vi "patientCreateView.vi"() -> ()   [LabVIEW 2019]
doc: "40"
uses:
  03_Home/controller/logoutBtn.ctl
  03_Home/controller/exitBtn.ctl
  <vilib>/Utility/miscctls.llb/LVPointTypeDef.ctl
  03_Home/controller/pannelState.ctl
  subVI/patients_state.ctl
  globalValue.vi
panel:
  in  "patients_weight":dbl format="%.1f"
  in  "patients_age":dbl
  in  "patients_height":dbl format="%.1f"
  in  "patients_birthdate":dbl format="%<%Y-%m-%d>T"
  in  "patients_gender":string(combo)
  in  "backPage":bool
  in  "patients_info":string
  in  "patients_address":string
  in  "patients_phone":string
  in  "patients_email":string
  in  "patients_nm":string
  in  "cancelBtn":bool
  in  "createBtn":bool
  out "patients_id":string
  in  "Help Button":bool
  in  "LogOut Button":T1
  in  "Exit Button":T2
  out "userNm":string
  # "|"
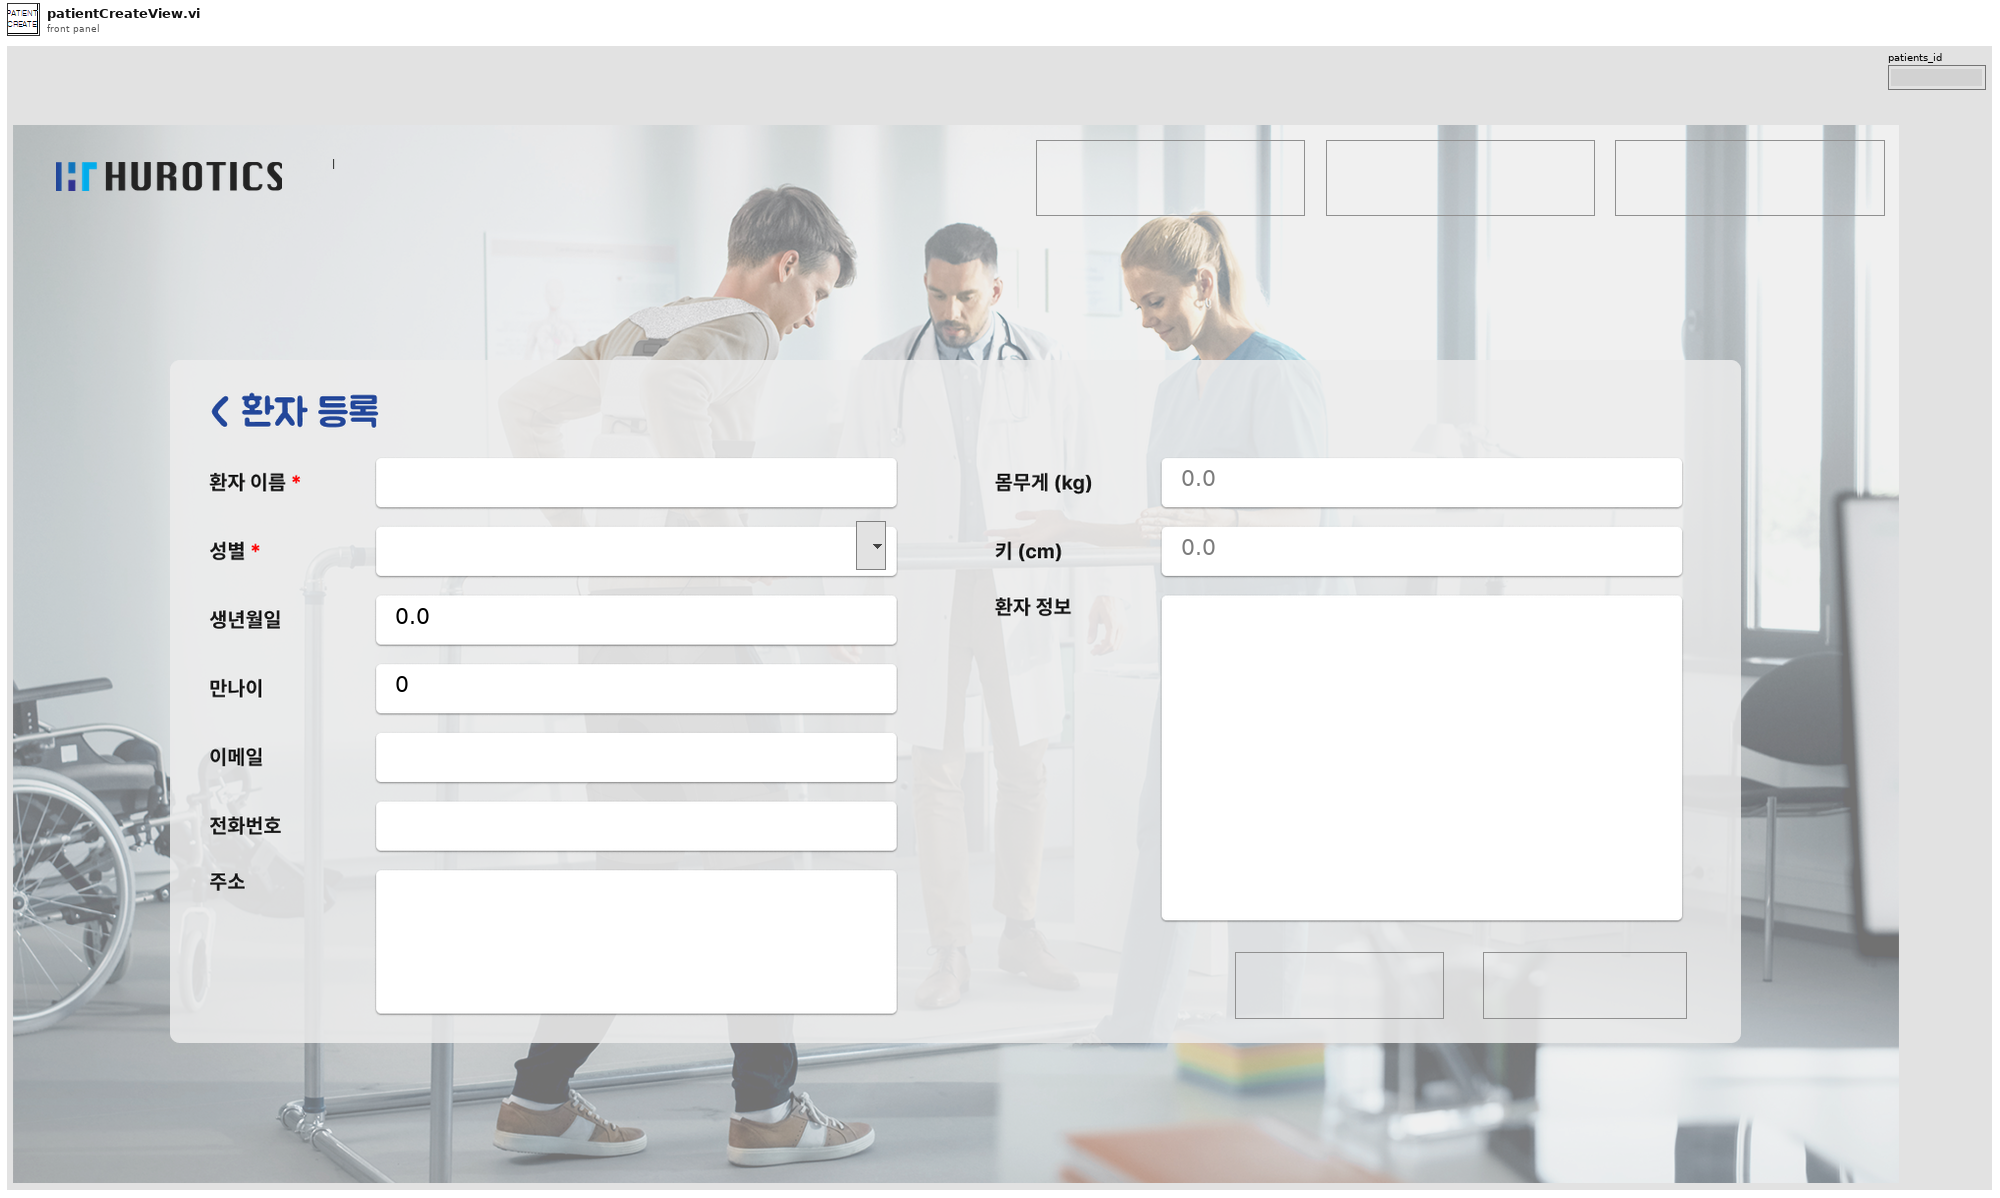
[diagram p1: front panel]
types:
  T1 = typedef "logoutBtn.ctl" = bool
  T2 = typedef "exitBtn.ctl" = bool
  T3 = typedef "LVPointTypeDef.ctl" = cluster{"Horizontal":i16, "Vertical":i16}
  T4 = enum16{"connection", "create", "getReadList", "getRead", "getCount", "update", "delete", "close"}
  T5 = typedef "pannelState.ctl" = enum16{"Init", "LogIn", "SignUpView", "Home", "Management_patientList", "Management_patientTrashtList", "Management_patientCreate", "Management_patientUpdate", "Management_patientTraining", "Management_patientTrainingDetail", "H-MEDI PatientList", "H-MEDI HardwareCtl", "Adjust", "FineTuning", "UserList", "UserDetail", "Exit"}
  T6 = typedef "patients_state.ctl" = enum16{"connection", "create", "getReadList", "getRead", "getCount", "update", "delete", "trash", "restore", "close"}
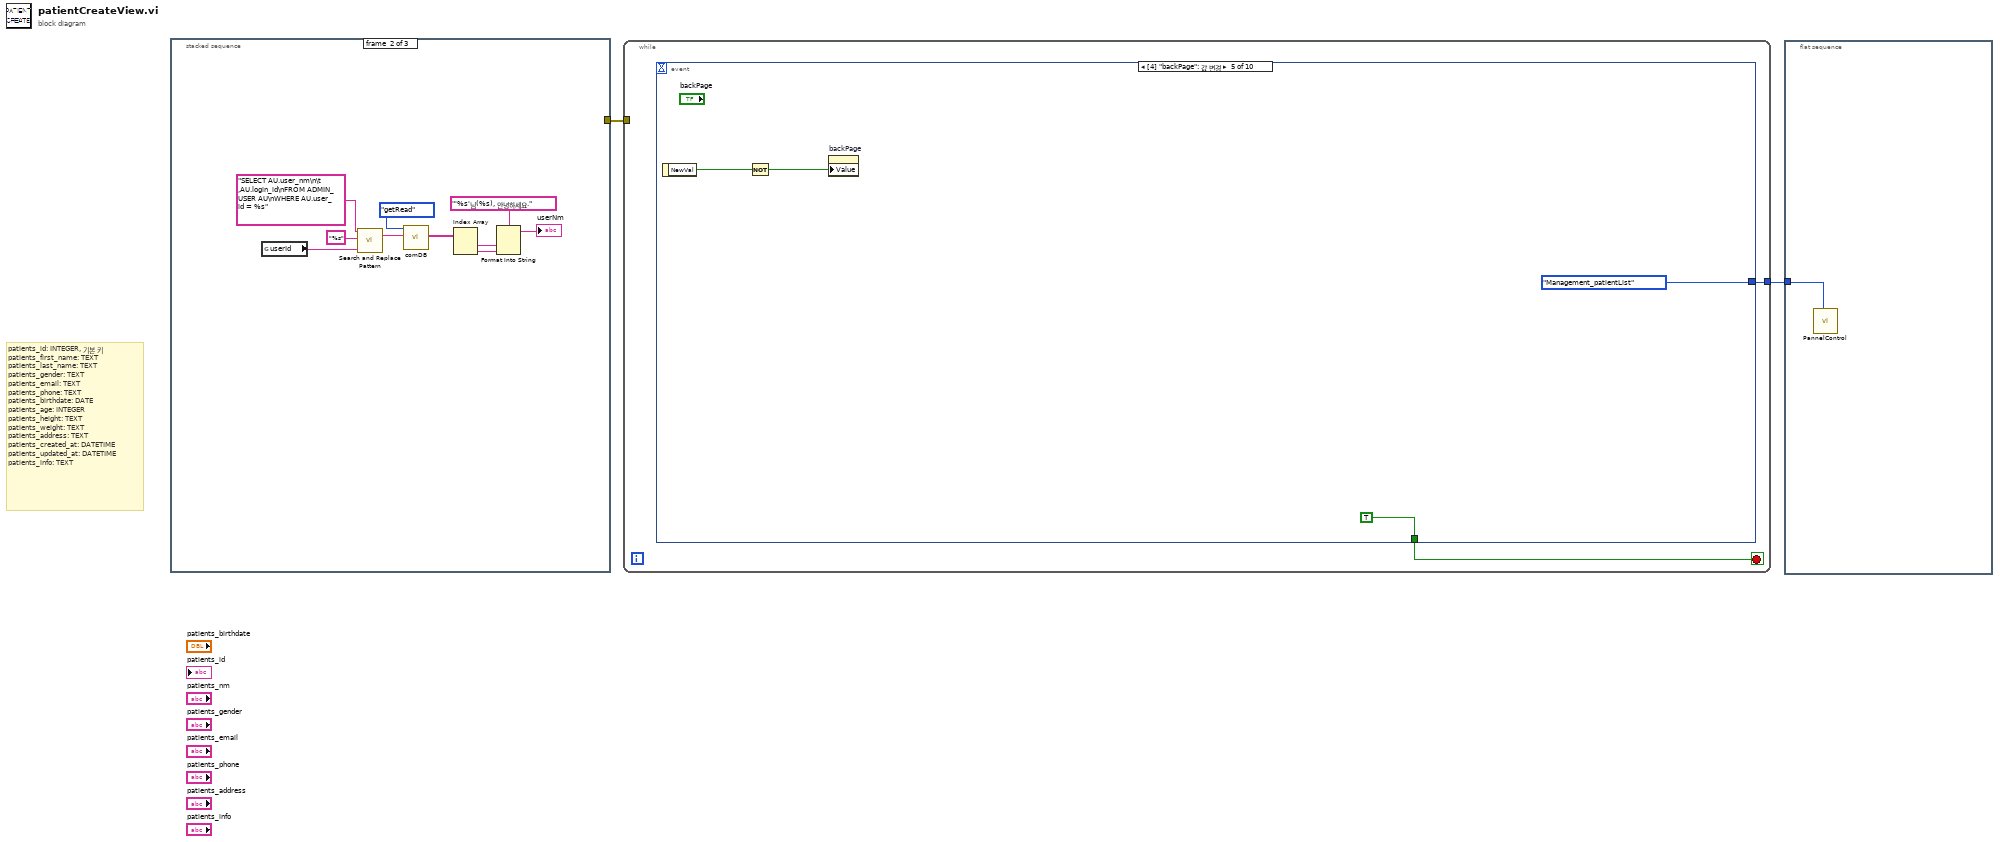
[diagram p0: block diagram]
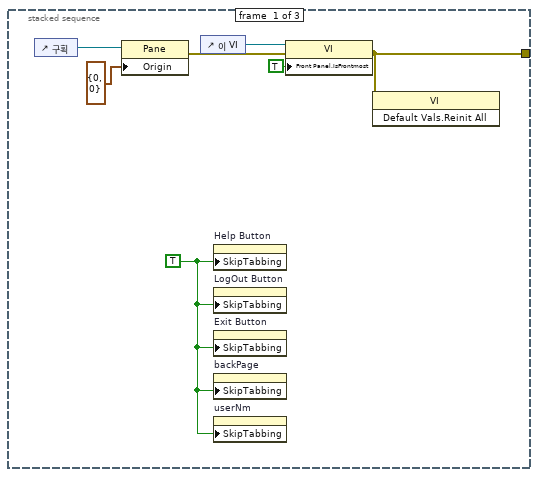
[diagram p2: hidden frame]
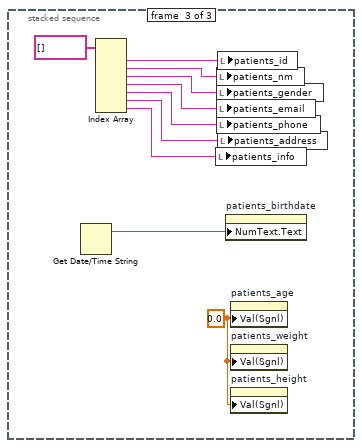
[diagram p3: hidden frame]
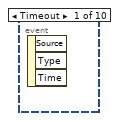
[diagram p4: hidden frame]
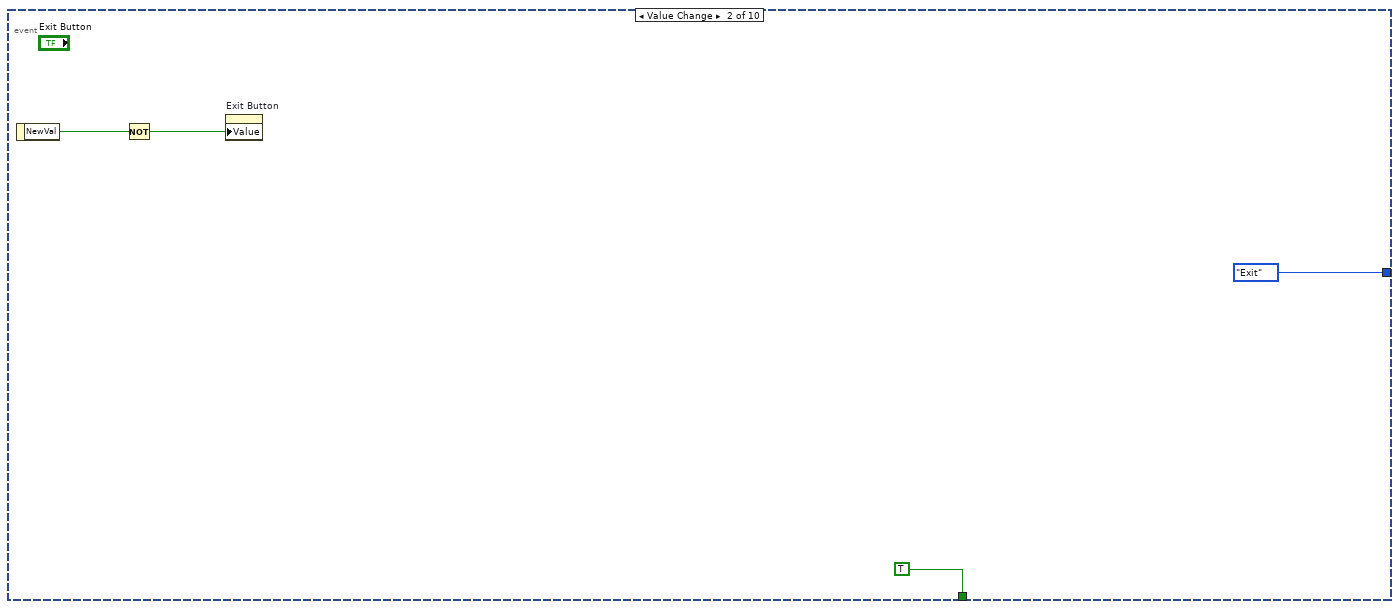
[diagram p5: hidden frame]
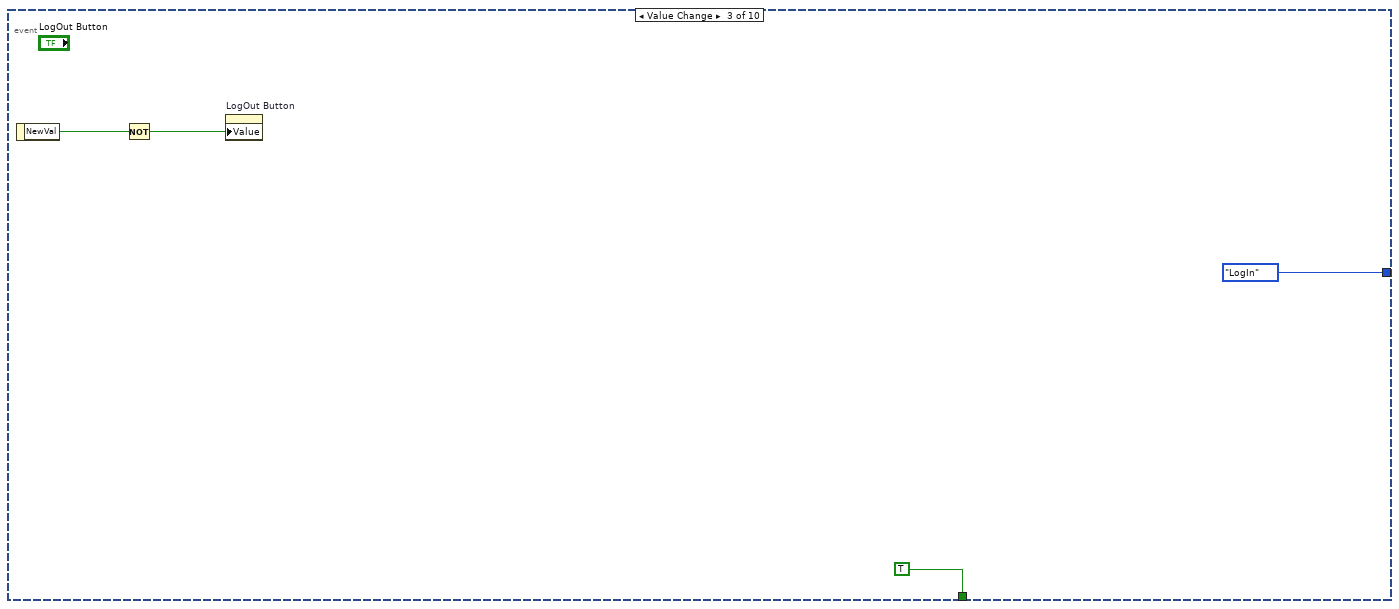
[diagram p6: hidden frame]
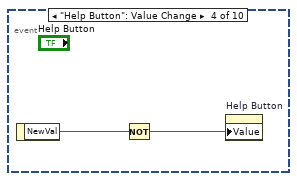
[diagram p7: hidden frame]
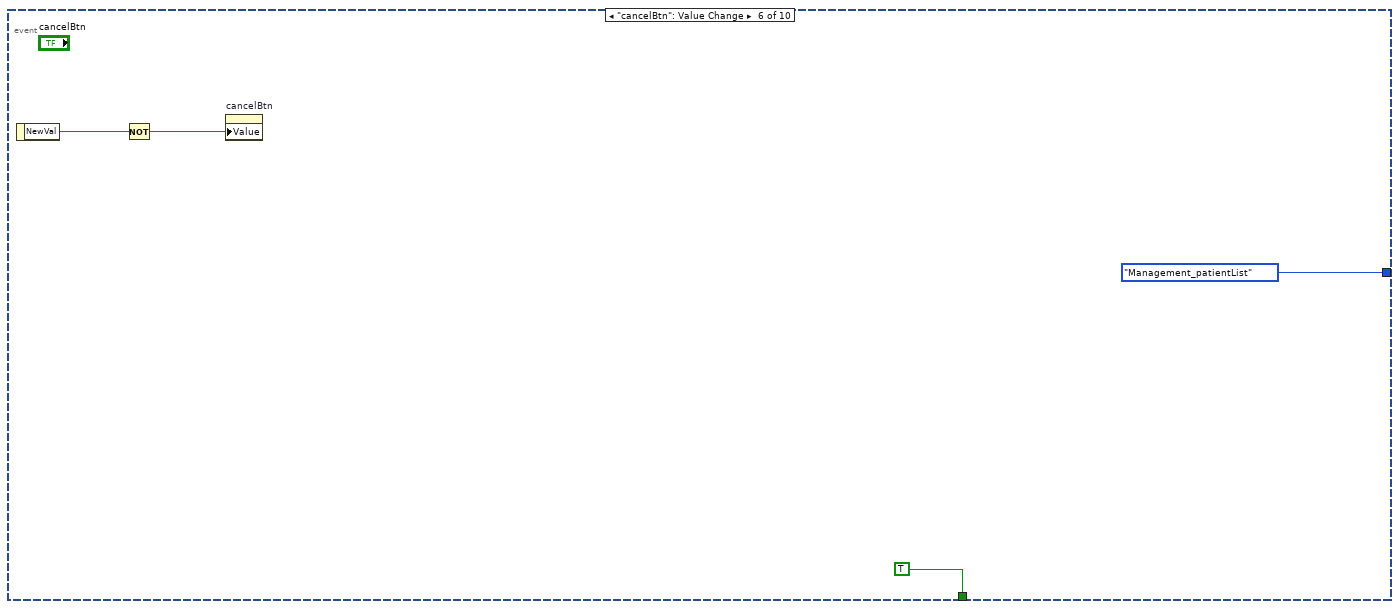
[diagram p8: hidden frame]
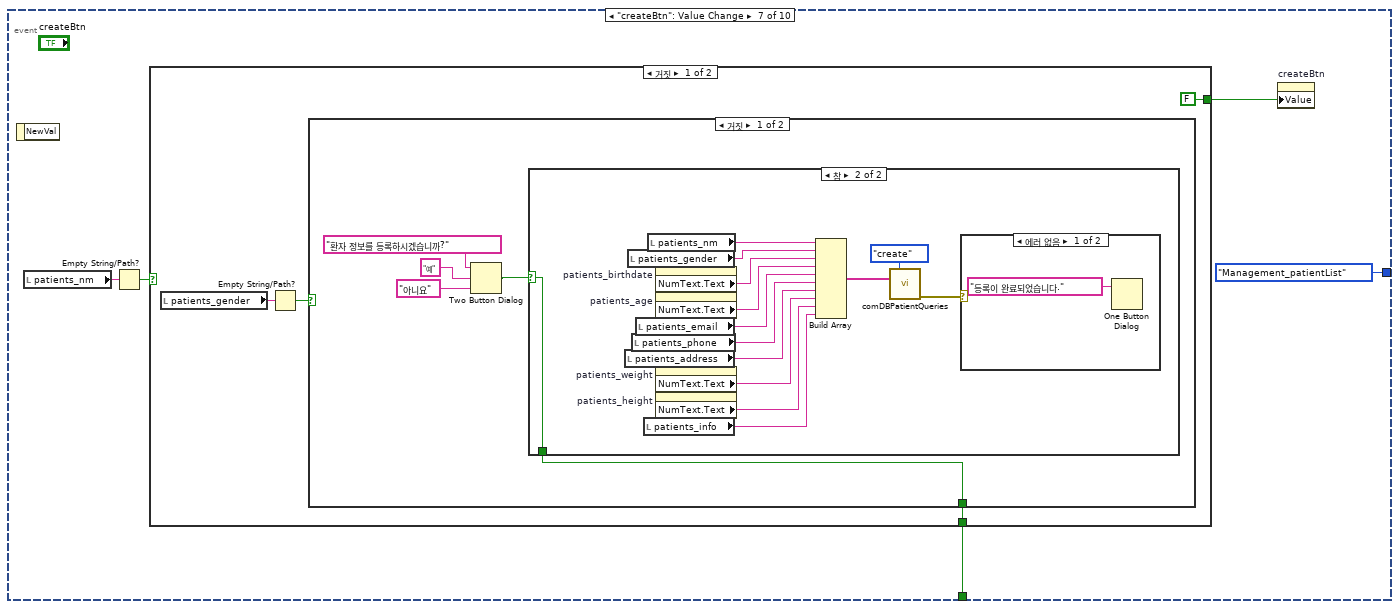
[diagram p9: hidden frame]
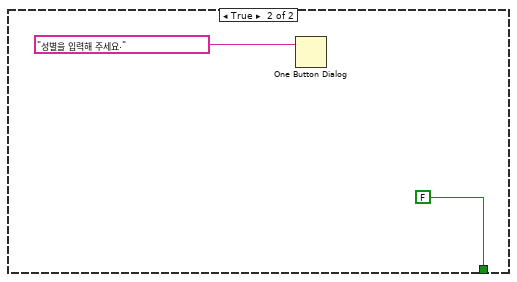
[diagram p12: hidden frame]
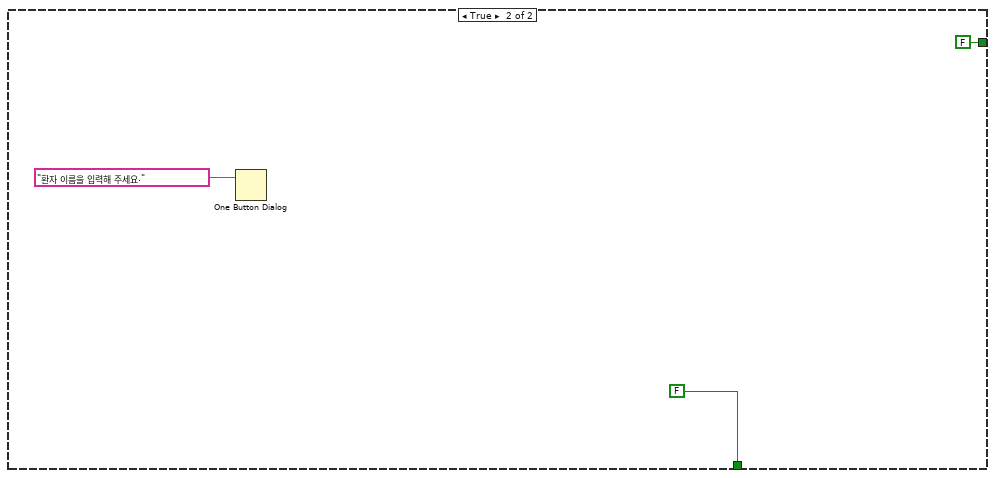
[diagram p13: hidden frame]
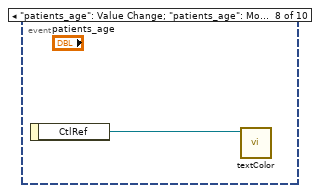
[diagram p14: hidden frame]
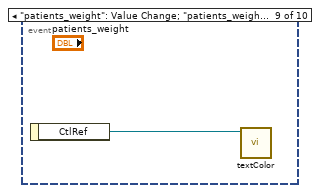
[diagram p15: hidden frame]
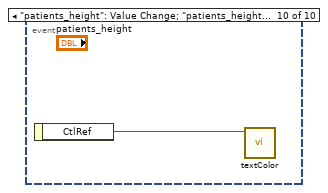
[diagram p16: hidden frame]
diagram:
  # "patients_id: INTEGER, 기본 키\npatients_first_name: TEXT\npatients_last_name: TEXT\npatients_gender: TEXT\npatients_email: TEXT\npatients_phone: TEXT\npatients_birthdate: DATE\npatients_age: INTEGER\npatients_height: TEXT\npatients_weight: TEXT\npatients_address: TEXT\npatients_created_at: DATETIME\npatients_updated_at: DATETIME\npatients_info: TEXT"
  n1 = stacked-sequence {
    tunnel: [w4 _ _] -> w1
    frame #0 {
      w3 = TRUE ("탭으로 이동 시 건너뛰기")
      n2 = control-ref of="구획"() -> (w7:refnum<vi>)
      n3 = property class="Pane"(reference=w7, "Origin"=T3 {"Horizontal"=0, "Vertical"=0} ("원점")) -> (error out=w5:errorcluster)  [unwired: 1 in, 1 out]
      n4 = control-ref of="이 VI"() -> (w9:refnum<vi>)
      n5 = property on="Help Button" class="Bool (엄격한)"("SkipTabbing"=w3) -> ()  [unwired: 2 in, 2 out]
      n6 = property on="LogOut Button" class="Bool (엄격한)"("SkipTabbing"=w3) -> ()  [unwired: 2 in, 2 out]
      n7 = property on="Exit Button" class="Bool (엄격한)"("SkipTabbing"=w3) -> ()  [unwired: 2 in, 2 out]
      n8 = property on="backPage" class="Bool (엄격한)"("SkipTabbing"=w3) -> ()  [unwired: 2 in, 2 out]
      n9 = property on="userNm" class="Str"("SkipTabbing"=w3) -> ()  [unwired: 2 in, 2 out]
      n10 = property class="VI"(reference=w9, error in=w5, "Front Panel.IsFrontmost"=TRUE ("프런트패널 윈도우:맨 앞으로")) -> (error out=w4:errorcluster)  [unwired: 1 out]
      n11 = invoke class="VI" method="Default Vals.Reinit All"(error in=w4) -> ()  [unwired: 2 in, 3 out]
    }
    frame #1 {
      n12 = global read "globalValue.vi" "userId"() -> (w10:string)
      n13 = call <vilib>:"Search and Replace Pattern.vi"("string"="SELECT AU.user_nm\n\t         ,AU.login_id\nFROM ADMIN_USER AU\nWHERE AU.user_id = %s" ("Query"), "regular expression (\"\")"="%s" ("regular expression (\"\")"), "replace string (\"\")"=w10) -> ("result string"=w11:string)  [unwired: 2 in, 1 out]
      n14 = call "comDB.vi"("Query"=w11, "State"=T4."getRead") -> ("result1DArray"=w17:string[])  [unwired: 5 in, 3 out]
      n15 = Index Array(array=w17) -> (element #1=w16:string, element #2=w15:string)  [unwired: 2 in]
      n16 = Format Into String(format string="'%s'님(%s), 안녕하세요." ("문자열"), w16, w15) -> (resulting string=→"userNm":string)  [unwired: 2 in, 1 out]
    }
    frame #2 {
      w21 = 0.0 ("값(신호)")
      n17 = Get Date/Time String() -> (date string=w20:string)  [unwired: 3 in, 1 out]
      n18 = Index Array(array=string[] [] ("배열")) -> (element #1=w28:string, element #2=w29:string, element #3=w27:string, element #4=w25:string, element #5=w24:string, element #6=w23:string, element #7=w22:string)  [unwired: 7 in]
      n19 = local write "patients_info"(w22) -> ()
      n20 = local write "patients_nm"(w29) -> ()
      n21 = local write "patients_gender"(w27) -> ()
      n22 = local write "patients_email"(w25) -> ()
      n23 = local write "patients_phone"(w24) -> ()
      n24 = local write "patients_id"(w28) -> ()
      n25 = local write "patients_address"(w23) -> ()
      n26 = property on="patients_birthdate" class="DigNum (엄격한)"("NumText.Text"=w20) -> ()  [unwired: 2 in, 2 out]
      n27 = property on="patients_age" class="DigNum (엄격한)"("Val(Sgnl)"=w21) -> ()  [unwired: 2 in, 2 out]
      n28 = property on="patients_weight" class="DigNum (엄격한)"("Val(Sgnl)"=w21) -> ()  [unwired: 2 in, 2 out]
      n29 = property on="patients_height" class="DigNum (엄격한)"("Val(Sgnl)"=w21) -> ()  [unwired: 2 in, 2 out]
    }
  }
  n30 = while {
    tunnel: [w30] -> w2
    tunnel: w1 -> [_]
    stop <- w31 stop-if-true
    n31 = event shown="[4] \"backPage\": 값 변경" {
      selector: _ -> [_ _ _ _ _ _ _ _ _ _]
      dyn-events: _ -> [_ _ _ _ _ _ _ _ _ _]
      timeout: _ -> [_ _ _ _ _ _ _ _ _ _]
      tunnel: [_ TRUE TRUE _ TRUE TRUE w51 _ _ _] -> w31
      tunnel: [_ pannelState."Exit" ("State") pannelState."LogIn" ("State") _ pannelState."Management_patientList" ("State") pannelState."Management_patientList" ("State") pannelState."Management_patientList" ("State") _ _ _] -> w30
      event Timeout {
        n32 = event-data() -> ()  [unwired: 1 in, 3 out]
      }
      event Value Change {
        n33 = event-data() -> ("NewVal"=w33:T2)  [unwired: 1 in]
        n34 = Not(x=w33) -> (.not. x?=w32:T2)
        n35 = property on="Exit Button" class="Bool (엄격한)"("Value"=w32) -> ()  [unwired: 2 in, 2 out]
      }
      event Value Change {
        n36 = event-data() -> ("NewVal"=w37:T1)  [unwired: 1 in]
        n37 = Not(x=w37) -> (.not. x?=w36:T1)
        n38 = property on="LogOut Button" class="Bool (엄격한)"("Value"=w36) -> ()  [unwired: 2 in, 2 out]
      }
      event "Help Button": Value Change {
        n39 = event-data() -> ("NewVal"=w41:bool)  [unwired: 1 in]
        n40 = Not(x=w41) -> (.not. x?=w40:bool)
        n41 = property on="Help Button" class="Bool (엄격한)"("Value"=w40) -> ()  [unwired: 2 in, 2 out]
      }
      event "backPage": Value Change {
        n42 = event-data() -> ("NewVal"=w44:bool)  [unwired: 1 in]
        n43 = Not(x=w44) -> (.not. x?=w43:bool)
        n44 = property on="backPage" class="Bool (엄격한)"("Value"=w43) -> ()  [unwired: 2 in, 2 out]
      }
      event "cancelBtn": Value Change {
        n45 = event-data() -> ("NewVal"=w49:bool)  [unwired: 1 in]
        n46 = Not(x=w49) -> (.not. x?=w48:bool)
        n47 = property on="cancelBtn" class="Bool (엄격한)"("Value"=w48) -> ()  [unwired: 2 in, 2 out]
      }
      event "createBtn": Value Change {
        n48 = event-data() -> ()  [unwired: 1 in, 1 out]
        n49 = local read "patients_nm"() -> (w54:string)
        n50 = Empty String/Path?(string/path=w54) -> (empty?=w53:bool)
        n51 = case shown="거짓" w53 {
          tunnel: [FALSE ("createBtn") FALSE ("createBtn")] -> w52
          tunnel: [w55 FALSE] -> w51
          frame False {
            n52 = local read "patients_gender"() -> (w58:string)
            n53 = Empty String/Path?(string/path=w58) -> (empty?=w57:bool)
            n54 = case shown="거짓" w57 {
              tunnel: [w59 FALSE] -> w55
              frame False {
                n55 = Two Button Dialog(message="환자 정보를 등록하시겠습니까?" ("메시지"), 1:"아니요" ("거짓 버튼 이름(\"취소\")"), 2:"예" ("참 버튼 이름(\"확인\")")) -> (T button?=w60:bool)
                n56 = case shown="참" w60 {
                  selector: w60 -> [w64 w69]
                  tunnel: [w64 w69] -> w59
                  frame False {
                  }
                  frame True {
                    n57 = local read "patients_address"() -> (w74:string)
                    n58 = local read "patients_gender"() -> (w71:string)
                    n59 = local read "patients_phone"() -> (w75:string)
                    n60 = local read "patients_email"() -> (w76:string)
                    n61 = local read "patients_info"() -> (w73:string)
                    n62 = local read "patients_nm"() -> (w77:string)
                    n63 = property on="patients_birthdate" class="DigNum (엄격한)"() -> ("NumText.Text"=w68:string)  [unwired: 2 in, 2 out]
                    n64 = property on="patients_age" class="DigNum (엄격한)"() -> ("NumText.Text"=w67:string)  [unwired: 2 in, 2 out]
                    n65 = property on="patients_weight" class="DigNum (엄격한)"() -> ("NumText.Text"=w66:string)  [unwired: 2 in, 2 out]
                    n66 = property on="patients_height" class="DigNum (엄격한)"() -> ("NumText.Text"=w65:string)  [unwired: 2 in, 2 out]
                    n67 = Build Array(w77, w71, w68, w67, w76, w75, w74, w66, w65, w73) -> (w72:string[])
                    n68 = call "comDBPatientQueries.vi"("State"=patients_state."create", "입력"=w72) -> ("error out"=w78:errorcluster)  [unwired: 10 in, 3 out]
                    n69 = case shown="에러 없음" w78 {
                      frame No Error {
                        n70 = One Button Dialog(message="등록이 완료되었습니다." ("메시지")) -> ()  [unwired: 1 in, 1 out]
                      }
                      frame Error {
                      }
                    }
                  }
                }
              }
              frame True {
                n71 = One Button Dialog(message="성별을 입력해 주세요." ("메시지")) -> ()  [unwired: 1 in, 1 out]
              }
            }
          }
          frame True {
            n72 = One Button Dialog(message="환자 이름을 입력해 주세요." ("메시지")) -> ()  [unwired: 1 in, 1 out]
          }
        }
        n73 = property on="createBtn" class="Bool (엄격한)"("Value"=w52) -> ()  [unwired: 2 in, 2 out]
      }
      event "patients_age": Value Change; "patients_age": Mouse Down {
        n74 = event-data() -> ("CtlRef"=w85:refnum<vi>)  [unwired: 1 in]
        n75 = call "textColor.vi"("디지털 입력"=w85) -> ()  [unwired: 11 in]
      }
      event "patients_weight": Value Change; "patients_weight": Mouse Down {
        n76 = event-data() -> ("CtlRef"=w86:refnum<vi>)  [unwired: 1 in]
        n77 = call "textColor.vi"("디지털 입력"=w86) -> ()  [unwired: 11 in]
      }
      event "patients_height": Value Change; "patients_height": Mouse Down {
        n78 = event-data() -> ("CtlRef"=w87:refnum<vi>)  [unwired: 1 in]
        n79 = call "textColor.vi"("디지털 입력"=w87) -> ()  [unwired: 11 in]
      }
    }
  }
  n80 = flat-sequence {
    tunnel: w2 -> [w88]
    frame #0 {
      n81 = call "PannelControl.vi"("State"=w88) -> ()  [unwired: 10 in, 1 out]
    }
  }
